vi "nirviWaitUntilNextMultiple.vi"(1 "Count(Ticks)":u32) -> (0 "Tick Count(Ticks)":u32)   [LabVIEW 2017]
doc: "Waits until the value of the timer becomes a multiple of <B>Count</B>. Use this function to synchronize activities. You can call this function in a loop to control the loop execution rate."
panel:
  in  "Counter Units":u16(ring) items=["Ticks", "uSec", "mSec"]
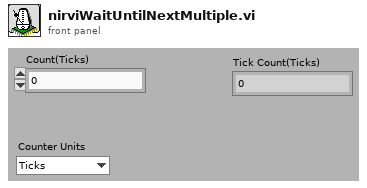
[diagram p1: front panel]
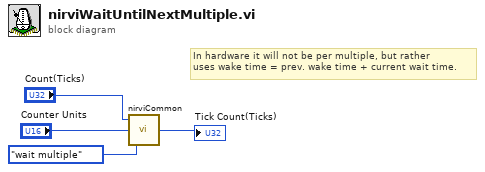
[diagram p0: block diagram]
diagram:
  # "In hardware it will not be per multiple, but rather\nuses wake time = prev. wake time + current wait time."
  n1 = call <vilib>:"nirviCommon.vi"("Action"=enum16{"wait", "wait multiple", "tick count"}."wait multiple", "Counter Units"="Counter Units", "Count(uSec)"="Count(Ticks)") -> ("Tick Count(uSec)"=→"Tick Count(Ticks)":u32)
